vi "Test Customer Status Updated On Submit Order.vi"(8 "error in (no error)":errorcluster, 11 "Customer Test in":refnum<class "Customer Test.lvclass">) -> (0 "error out":errorcluster, 3 "Customer Test out":refnum<class "Customer Test.lvclass">)   [LabVIEW 2020, in "Customer Test.lvclass"]
uses:
  Customer Test.lvclass
  C:/Program Files (x86)/National Instruments/LabVIEW 2020/vi.lib/Astemes/LUnit/Test Case.lvclass
  Processes/People/Customers/Customer/Customer.lvclass
  C:/Program Files (x86)/National Instruments/LabVIEW 2020/vi.lib/Astemes/Triarc Framework/Process/Process.lvclass
  Support/Beverages/TypeDefs/Drink Type.ctl
  Support/Beverages/TypeDefs/Options.ctl
  Test Doubles/Stub Job Handler/Stub Job Handler.lvclass
  C:/git/astemes-triarc-examples/source/Coffee Shop/Processes/People/Process Job/Job Handler.lvclass
  <vilib>/Astemes/Triarc Framework/Process/Process.lvclass/Process.ctl
  <vilib>/Astemes/LUnit/Test Case.lvclass/Test Case.ctl
  <vilib>/Astemes/Triarc Framework/Process/Public/Lifecycle/Get Lifecycle State.vi
  <vilib>/Astemes/Triarc Framework/Broadcast Event Helpers/Execution timer.vi
  <vilib>/Astemes/Triarc Framework/Process/Private/SubVIs/Wait for finish.vi
  <vilib>/Astemes/Triarc Framework/Process/Private/SubVIs/Set Lifecycle State.vi
  <vilib>/Astemes/Triarc Framework/Process/Protected/Messaging/Send Message.vi
  <vilib>/Astemes/LUnit/Append Pass Result.vi
  <vilib>/Astemes/LUnit/Append Fail Result.vi
  <vilib>/Utility/error.llb/Clear Errors.vi
  <vilib>/Astemes/Triarc Framework/Process/Private/SubVIs/Handle Debug Data.vi
  <vilib>/Astemes/Triarc Framework/Logging/Log Debug.vi
  <vilib>/AdvancedString/1D String Array to Delimited String.vi
  <vilib>/Utility/High Resolution Relative Seconds.vi
  <vilib>/Utility/error.llb/Error Cluster From Error Code.vi
  <vilib>/Astemes/Triarc Framework/Support/Dequeue Broadcast Message.vi
  <vilib>/Astemes/Triarc Framework/Process/Public/Read Name.vi
  <vilib>/Astemes/Triarc Framework/Callback/Callback.lvclass
  <vilib>/Astemes/Triarc Framework/Process/Process.lvclass
  Customer Test.lvclass/Customer Test.ctl
  Support/Beverages/Beverage/Beverage.lvclass
  <vilib>/Astemes/LUnit/Test Case.lvclass
  <vilib>/Astemes/Triarc Framework/Support/Broadcast Event Dequeuers.lvlib
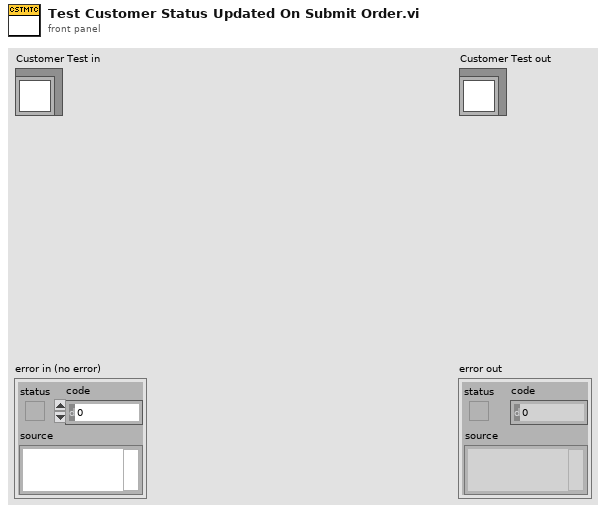
[diagram p1: front panel]
types:
  T1 = typedef "Beverage.lvclass/Drink Type.ctl" = enum16{"Dark Roast", "Decaf", "Espresso", "House Blend"}
  T2 = typedef "Beverage.lvclass/Options.ctl" = enum16{"<None>", "Milk", "Mocha", "Soy", "Whip"}
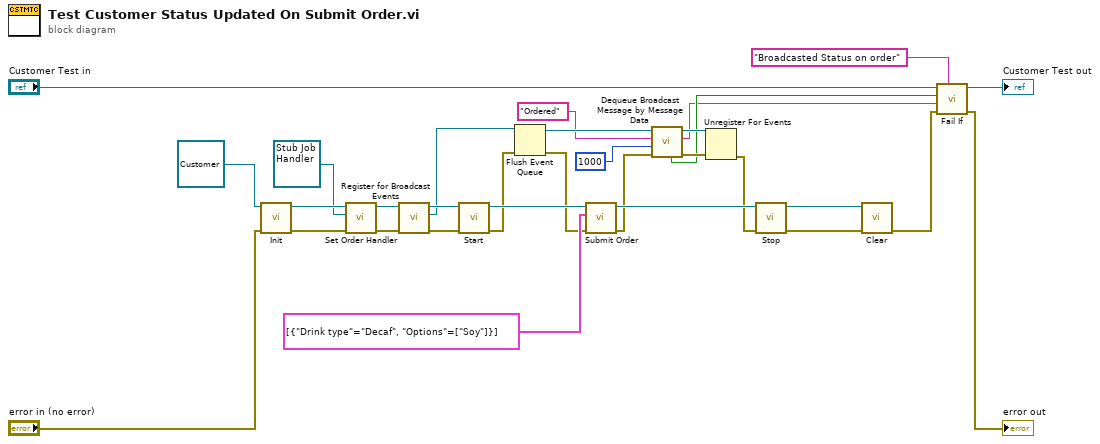
[diagram p0: block diagram]
diagram:
  n1 = call-dynamic "Init.vi"("error in (no error)"="error in (no error)", "View In"=refnum<class "Customer.lvclass"> refnum ("Customer.lvclass")) -> ("error out"=w28:errorcluster, "View Out"=w11:refnum<class "Customer.lvclass">)  [unwired: 8 in]
  n2 = call "Set Order Handler.vi"("error in (no error)"=w28, "Order Handler"=refnum<class "Stub Job Handler.lvclass"> refnum ("Stub Job Handler.lvclass"), "Customer In"=w11) -> ("error out"=w12:errorcluster, "Customer Out"=w10:refnum<class "Customer.lvclass">)  [unwired: 7 in]
  n3 = call <vilib>:"Register for Broadcast Events.vi"("error in (no error)"=w12, "Process In"=w10) -> ("error out"=w30:errorcluster, "Event Registration Refnum Out"=w13:refnum<event-registration>, "Process Out"=w29:refnum<class "Customer.lvclass">)  [unwired: 7 in]
  n4 = call <vilib>:"Start.vi"("error in (no error)"=w30, "Process In"=w29) -> ("error out"=w22:errorcluster, "Process Out"=w24:refnum<class "Customer.lvclass">)  [unwired: 7 in, 1 out]
  n5 = Flush Event Queue(0:w13, 3:w22) -> (8:w8:refnum<event-registration>, 11:w14:errorcluster)  [unwired: 4 in, 1 out]
  n6 = call "Submit Order.vi"("error in (no error)"=w14, "Order Content"=cluster{"Drink type":T1, "Options":T2[]}[] [{"Drink type"=enum."Decaf", "Options"=[enum."Soy"]}] ("Order"), "Customer In"=w24) -> ("error out"=w5:errorcluster, "Customer Out"=w23:refnum<class "Customer.lvclass">)  [unwired: 7 in]
  n7 = call <vilib>:"Dequeue Broadcast Message by Message Data.vi"("error in (no error)"=w5, "Timeout (-1)"=1000, "Message Data"="Ordered" ("Message"), "Event Registration Refnum"=w8) -> ("error out"=w6:errorcluster, "Message"=w1:string, "Event Registration Refnum Out"=w7:refnum<event-registration>, "Timed Out?"=w2:bool)  [unwired: 3 in, 1 out]
  n8 = Unregister For Events(event registration refnum=w7, error in=w6) -> (error out=w19:errorcluster)
  n9 = call <vilib>:"Stop.vi"("error in (no error)"=w19, "Process In"=w23) -> ("error out"=w26:errorcluster, "Process Out"=w27:refnum<class "Customer.lvclass">)  [unwired: 7 in, 1 out]
  n10 = call-dynamic "Clear.vi"("error in (no error)"=w26, "View In"=w27) -> ("error out"=w18:errorcluster)  [unwired: 9 in]
  n11 = call <vilib>:"Fail If.vi"("Description"="Broadcasted Status on order", "error in (no error)"=w18, "Message"=w1, "Fail?"=w2, "LUnit Test Case In"="Customer Test in") -> ("error out"=→"error out":errorcluster, "LUnit Test Case Out"=→"Customer Test out":refnum<class "Customer Test.lvclass">)  [unwired: 5 in]
